vi "Main Page VI Name.vi"(11 "CD Template in":refnum<class "NIVS_Asynchronous.lvclass">) -> (2 "Main Page VI Name":string)   [LabVIEW 2023, in "NIVS_Asynchronous.lvclass"]
uses:
  NIVS_Asynchronous.lvclass
  NIVS_Asynchronous.lvclass/NIVS_Asynchronous.ctl
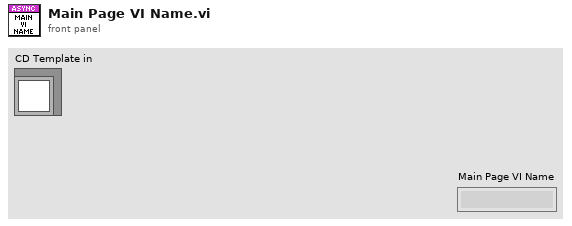
[diagram p1: front panel]
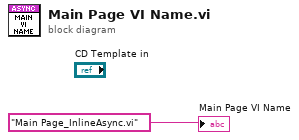
[diagram p0: block diagram]
diagram:
  "Main Page VI Name" <- "Main Page_InlineAsync.vi" ("Main Page VI Name")
